vi "Read Controls refs.vi"(8 "error in (no error)":errorcluster, 11 "Detector in":refnum<class "Detector.lvclass">) -> (0 "error out":errorcluster, 2 "Controls refs":T1 {"ref h5_file" format="%.0x"}, 3 "Detector out":refnum<class "Detector.lvclass">)   [LabVIEW 2020, in "Detector.lvclass"]
uses:
  Detector.lvclass
  Controls-refs_CLIENT.ctl
  <vilib>/addons/h5labview2/base/hid_t.ctl
  Detector.lvclass/Detector.ctl
  Control/Control-Client/Control-Client.lvclass
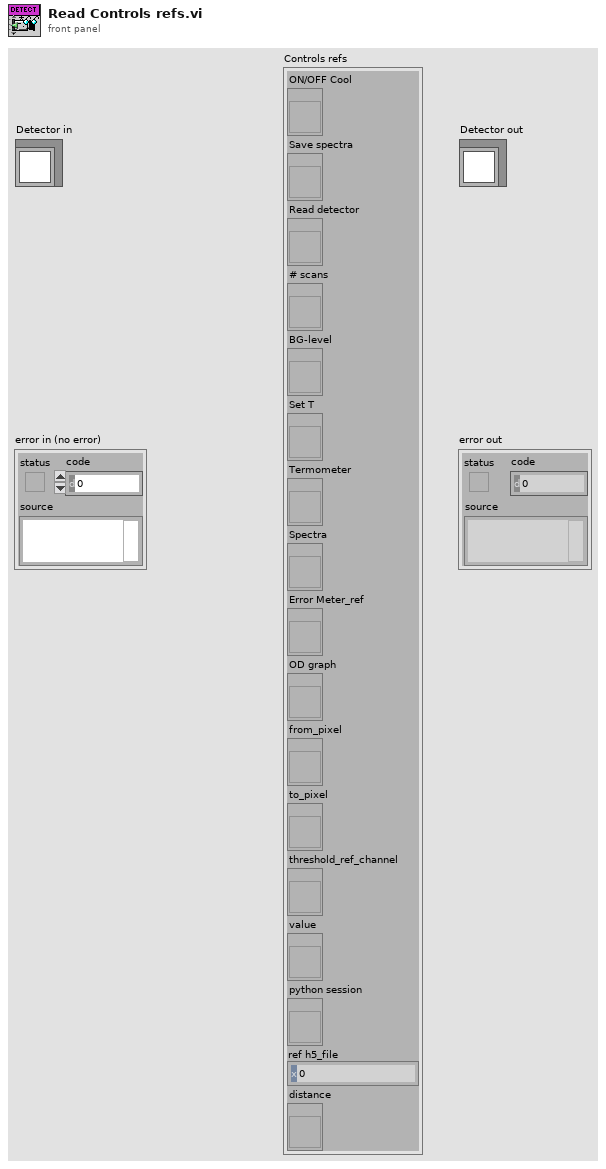
[diagram p1: front panel]
types:
  T1 = typedef "Control-Client.lvclass/Controls-refs_CLIENT.ctl" = cluster{"ON/OFF Cool":refnum<vi>, "Save spectra":refnum<vi>, "Read detector":refnum<vi>, "# scans":refnum<vi>, "BG-level":refnum<vi>, "Set T":refnum<vi>, "Termometer":refnum<vi>, "Spectra":refnum<vi>, "Error Meter_ref":refnum<vi>, "OD graph":refnum<vi>, "from_pixel":refnum<vi>, "to_pixel":refnum<vi>, "threshold_ref_channel":refnum<vi>, "value":refnum<vi>, "python session":refnum<vi>, "ref h5_file":T2, "distance":refnum<vi>}
  T2 = typedef "hid_t.ctl" = i64
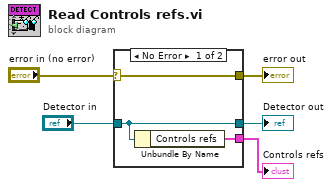
[diagram p0: block diagram]
diagram:
  n1 = case shown="No Error" "error in (no error)" {
    selector: "error in (no error)" -> [w8 w9]
    tunnel: [w8 w9] -> w4
    tunnel: [w7 w10] -> w2
    tunnel: "Detector in" -> [w7 w10]
    tunnel: [w6 _] -> w1
    frame No Error {
      n2 = Unbundle By Name(w7) -> ("Controls refs"=w6:T1)
    }
    frame Error {
    }
  }
  "error out" <- w4
  "Detector out" <- w2
  "Controls refs" <- w1
